vi "Cycle.vi"(8 "error in (no error)":errorcluster, 11 "MouseMultiDim In":refnum<class "MouseMultiDim.lvclass">) -> (0 "error out":errorcluster, 3 "MouseMultiDim Out":refnum<class "MouseMultiDim.lvclass">)   [LabVIEW 2012, in "MouseMultiDim.lvclass"]
uses:
  MouseMultiDim.lvclass
  Trial Based Experiment Statechart/PassiveExperiment/PassiveExperiment.lvclass
panel:
  out "ExperimentStats":T1
  in  "FixationRadius 2":dbl=34.0
  in  "RewardAmount 2":dbl=50.0
  out "Timeouts":T2={"Intertrial"=1500.0, "AcquireFixation"=4000.0, "HoldFixation"=300.0, "DelayPeriod"=2000.0, "ResponsePeriod"=0.0}
  in  "Eye Params 2":dbl[](array[numeric])
  out "XY Graph 2":cluster{"horizontal":dbl[], "vertical":dbl[]}[](graph)
  out "Elapsed Time (s)":dbl
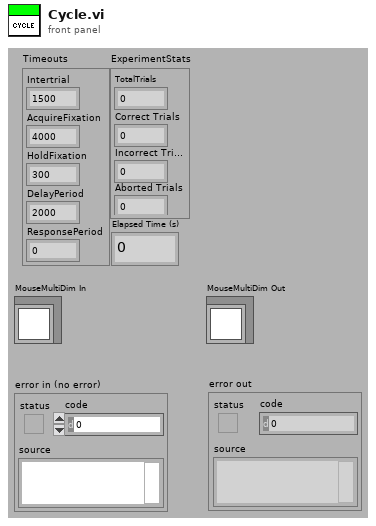
[diagram p1: front panel]
types:
  T1 = cluster{"TotalTrials":dbl, "Correct Trials":dbl, "Incorrect Trials":dbl, "Aborted Trials":dbl}
  T2 = cluster{"Intertrial":dbl, "AcquireFixation":dbl, "HoldFixation":dbl, "DelayPeriod":dbl, "ResponsePeriod":dbl}
  T3 = cluster{"TotalTrials":u32, "Correct Trials":u32, "Incorrect Trials":u32, "Aborted Trials":u32}
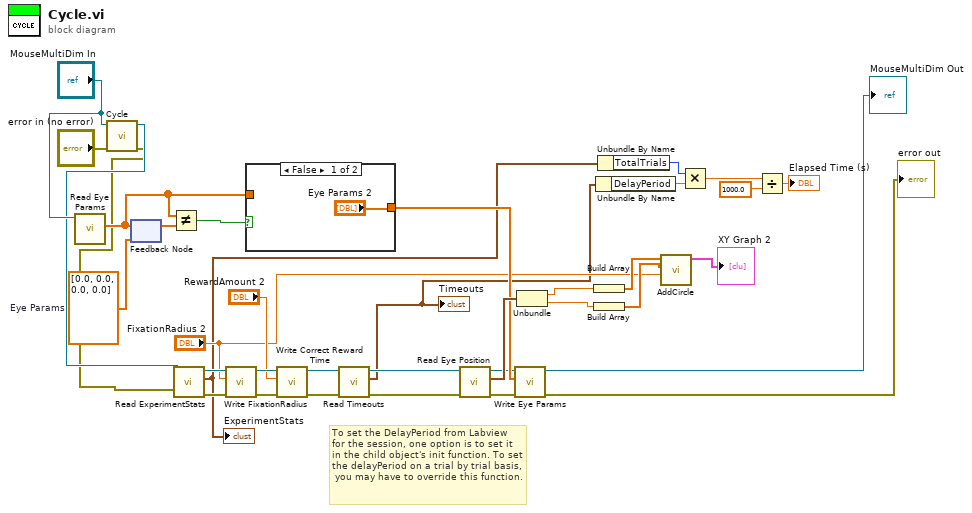
[diagram p0: block diagram]
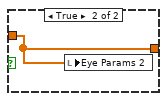
[diagram p2: hidden frame]
diagram:
  w30 = dbl[] [0.0, 0.0, 0.0, 0.0]  # Eye Params
  # "To set the DelayPeriod from Labview\nfor the session, one option is to set it \nin the child object's init function. To set\nthe delayPeriod on a trial by trial basis,\n you may have to override this function."
  n1 = call-dynamic "Read Eye Params.vi"("TrialBasedExperiment in"="MouseMultiDim In") -> ("Eye Params"=w31:dbl[])  [unwired: 8 in, 2 out]
  n2 = call-parent "Cycle.vi"("error in (no error)"="error in (no error)", "PassiveExperiment In"="MouseMultiDim In") -> ("error out"=w3:errorcluster, "PassiveExperiment Out"=w4:refnum<class "MouseMultiDim.lvclass">)  [unwired: 8 in]
  n3 = feedback #1(w30) -> (w28:dbl[])
  n4 = feedback-in #1(w31) -> ()
  n5 = Not Equal?(x=w31, y=w28) -> (x != y?=w29:bool)
  n6 = call-dynamic "Read ExperimentStats.vi"("error in (no error)"=w3, "TrialBasedExperiment in"=w4) -> ("error out"=w21:errorcluster, "ExperimentStats"=w7:T3, "TrialBasedExperiment out"=w20:refnum<class "MouseMultiDim.lvclass">)  [unwired: 7 in]
  "ExperimentStats" <- w7
  n7 = call-dynamic "Write FixationRadius.vi"("error in (no error)"=w21, "FixationRadius"="FixationRadius 2", "MatlabExperiment in"=w20) -> ("error out"=w24:errorcluster, "MatlabExperiment out"=w23:refnum<class "MouseMultiDim.lvclass">)  [unwired: 7 in]
  n8 = case shown="False" w29 {
    tunnel: ["Eye Params 2" w38] -> w34
    tunnel: w31 -> [_ w38]
    frame False {
    }
    frame True {
      n9 = local write "Eye Params 2"(w38) -> ()
    }
  }
  n10 = call-dynamic "Write Correct Reward Time.vi"("error in (no error)"=w24, "Correct Reward Time"="RewardAmount 2", "MatlabExperiment in"=w23) -> ("error out"=w26:errorcluster, "MatlabExperiment out"=w25:refnum<class "MouseMultiDim.lvclass">)  [unwired: 7 in]
  n11 = call-dynamic "Read Timeouts.vi"("error in (no error)"=w26, "TrialBasedExperiment in"=w25) -> ("error out"=w27:errorcluster, "Timeouts"=w6:T2, "TrialBasedExperiment out"=w13:refnum<class "MouseMultiDim.lvclass">)  [unwired: 7 in]
  "Timeouts" <- w6
  n12 = call-dynamic "Read Eye Position.vi"("error in (no error)"=w27, "TrialBasedExperiment in"=w13) -> ("error out"=w33:errorcluster, "Eye Position"=w35:cluster{"Horizontal":dbl, "Vertical":dbl}, "TrialBasedExperiment out"=w32:refnum<class "MouseMultiDim.lvclass">)  [unwired: 7 in]
  n13 = call-dynamic "Write Eye Params.vi"("error in (no error)"=w33, "Eye Params"=w34, "TrialBasedExperiment in"=w32) -> ("error out"=→"error out":errorcluster, "TrialBasedExperiment out"=→"MouseMultiDim Out":refnum<class "MouseMultiDim.lvclass">)  [unwired: 7 in]
  n14 = Unbundle(w35) -> ("Horizontal"=w19:dbl, "Vertical"=w18:dbl)
  n15 = Build Array(w19) -> (w17:dbl[])
  n16 = Build Array(w18) -> (w16:dbl[])
  n17 = Unbundle By Name(w6) -> ("DelayPeriod"=w9:dbl)
  n18 = Unbundle By Name(w7) -> ("TotalTrials"=w10:u32)
  n19 = call "AddCircle.vi"("radius"="FixationRadius 2", "vertical"=w16, "horizontal"=w17) -> ("output"=→"XY Graph 2":cluster{"horizontal":dbl[], "vertical":dbl[]}[])  [unwired: 8 in]
  n20 = Multiply(x=w10, y=w9) -> (x*y=w12:dbl)
  n21 = Divide(x=w12, y=1000.0) -> (x/y=→"Elapsed Time (s)":dbl)
